vi "FTA10-1000 Sum.vi"(11 "In":string) -> (1 "Lsum_String":string, 2 "Lsum":u8 format="%x", 3 "Out":string)   [LabVIEW 2018]
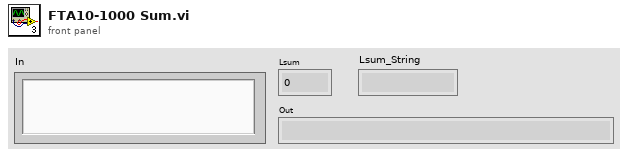
[diagram p1: front panel]
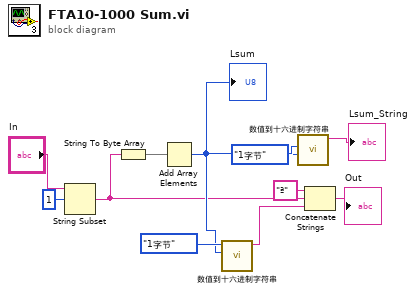
[diagram p0: block diagram]
diagram:
  n1 = String Subset(string="In", offset (0)=1 ("偏移量(0)")) -> (substring=w3:string)  [unwired: 1 in]
  n2 = String To Byte Array(string=w3) -> (unsigned byte array=w11:u8[])
  n3 = Add Array Elements(numeric array=w11) -> (sum=w7:u8)
  "Lsum" <- w7
  n4 = call "数值到十六进制字符串.vi"("Numeric"=w7, "转换字节数"=enum16{"1字节", "2字节", "4字节", "3字节"}."1字节") -> ("转换结果"=w9:string)  [unwired: 8 in, 1 out]
  n5 = call "数值到十六进制字符串.vi"("Numeric"=w7, "转换字节数"=enum16{"1字节", "2字节", "4字节", "3字节"}."1字节") -> ("转换结果"=→"Lsum_String":string)  [unwired: 8 in, 1 out]
  n6 = Concatenate Strings("ª" ("字符串"), w3, w9) -> (→"Out":string)
